vi "Generator Driver Template 5.vi"() -> ()   [LabVIEW 2024]
uses:
  <vilib>/addons/control/pid/pid.llb/PID (DBL).vi
  subVIs/Revidyne Generator.lvlib
  <vilib>/addons/control/pid/NI_PID_pid.lvlib
  <vilib>/ptbypt/NI_PtbyPt.lvlib
panel:
  in  "Low":dbl(slide) scale=0.0..255.0
  in  "High":dbl(slide) scale=0.0..255.0
  in  "PID gains":T1={"proportional gain (Kc)"=1.0, "integral time (Ti, min)"=0.01, "derivative time (Td, min)"=0.0} {"derivative time (Td, min)" format="%.3f"; "integral time (Ti, min)" format="%.3f"; "proportional gain (Kc)" format="%.3f"}
  in  "Load":dbl(slide) scale=0.0..1000.0
  out "Waveform Chart":cluster{"Value":dbl, "output":dbl}(graph)
  in  "Speed":dbl(slide) scale=0.0..255.0
  in  "stop":bool
  in  "VISA resource name":refnum<visa-resource-name>
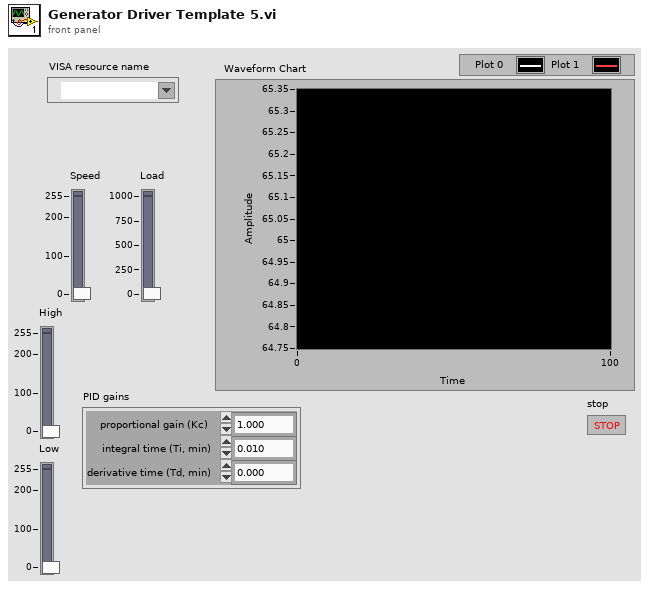
[diagram p1: front panel]
types:
  T1 = cluster{"proportional gain (Kc)":dbl, "integral time (Ti, min)":dbl, "derivative time (Td, min)":dbl}
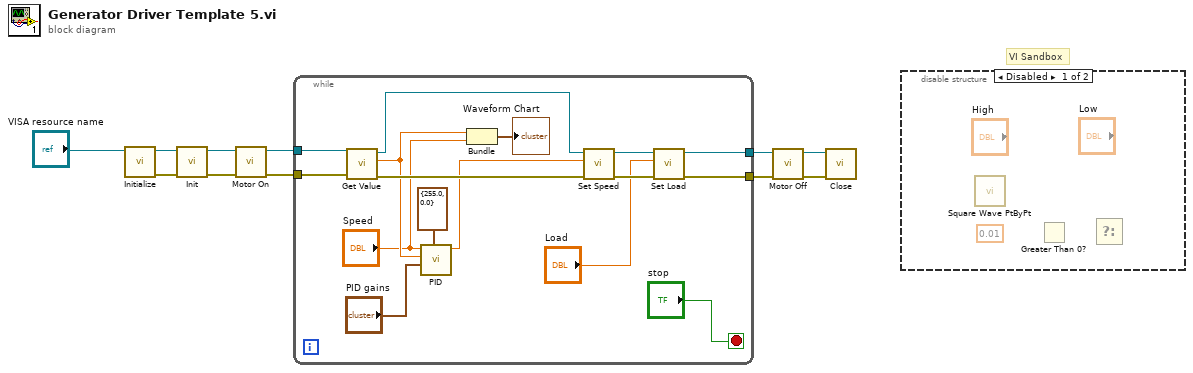
[diagram p0: block diagram]
diagram:
  # "VI Sandbox"
  n1 = call "Initialize.vi"("VISA resource name"="VISA resource name") -> ("error out"=w10:errorcluster, "VISA resource name out"=w11:refnum<visa-resource-name>)  [unwired: 9 in]
  n2 = call "Init.vi"("error in (no error)"=w10, "VISA resource name"=w11) -> ("error out"=w8:errorcluster, "VISA resource name out"=w9:refnum<visa-resource-name>)  [unwired: 8 in]
  n3 = call "Motor On.vi"("error in"=w8, "VISA resource name"=w9) -> ("error out"=w6:errorcluster, "VISA resource name out"=w7:refnum<visa-resource-name>)  [unwired: 8 in]
  n4 = while {
    tunnel: w7 -> [w27]
    tunnel: w6 -> [w26]
    tunnel: [w19] -> w4
    tunnel: [w20] -> w1
    stop <- "stop" stop-if-true
    n5 = call "Get Value.vi"("error in (no error)"=w26, "VISA resource name"=w27) -> ("error out"=w24:errorcluster, "Value"=w15:dbl, "VISA resource name out"=w23:refnum<visa-resource-name>)  [unwired: 7 in]
    n6 = call-poly <vilib>:"PID.vi"("output range"=cluster{"output high":dbl, "output low":dbl} {"output high"=255.0, "output low"=0.0}, "PID gains"="PID gains", "process variable"=w15, "setpoint"="Speed") -> ("output"=w13:dbl)  [unwired: 6 in, 1 out]
    n7 = Bundle("Value"=w15, "Speed"="Speed") -> (→"Waveform Chart":cluster{"Value":dbl, "Speed":dbl})  [unwired: 1 in]
    n8 = call "Set Speed.vi"("error in (no error)"=w24, "speed (0)"=w13, "VISA resource name"=w23) -> ("error out"=w21:errorcluster, "VISA resource name out"=w22:refnum<visa-resource-name>)  [unwired: 7 in]
    n9 = call "Set Load.vi"("error in (no error)"=w21, "load (0)"="Load", "VISA resource name"=w22) -> ("error out"=w19:errorcluster, "VISA resource name out"=w20:refnum<visa-resource-name>)  [unwired: 7 in]
  }
  n10 = call "Motor Off.vi"("error in (no error)"=w4, "VISA resource name"=w1) -> ("error out"=w3:errorcluster, "VISA resource name out"=w5:refnum<visa-resource-name>)  [unwired: 8 in]
  n11 = call "Close.vi"("error in (no error)"=w3, "VISA resource name"=w5) -> ()  [unwired: 9 in, 1 out]
  n12 = disable-structure shown="Disabled" {
    frame Disabled {
      (unwired) 0.01 ("frequency")
      n13 = call <vilib>:"Square Wave PtByPt.vi"() -> ()  [unwired: 5 in, 1 out]
      n14 = Greater Than 0?() -> ()  [unwired: 1 in, 1 out]
      n15 = Select() -> ()  [unwired: 3 in, 1 out]
    }
    frame Enabled {
    }
  }
